vi "AMZ_S3_APIHLP_Parse Setup Bucket Notification Request Parameters.vi"(8 "error in (no error)":errorcluster, 11 "Setup Notification Request parameters":T1) -> (0 "error out":errorcluster, 5 "PUT Data":string)   [LabVIEW 2015, in "LV Interface for Amazon S3.lvlib"]
uses:
  LV Interface for Amazon S3.lvlib
  Typedefs/AMZ_S3_NotificationConfiguration.ctl
  Typedefs/AMZ_S3_CompleteTopicConfiguration.ctl
  Typedefs/AMZ_S3_Event.ctl
  Typedefs/AMZ_S3_FilterRule.ctl
  Typedefs/AMZ_S3_CloudFunctionConfiguration.ctl
  Typedefs/AMZ_S3_QueueConfiguration.ctl
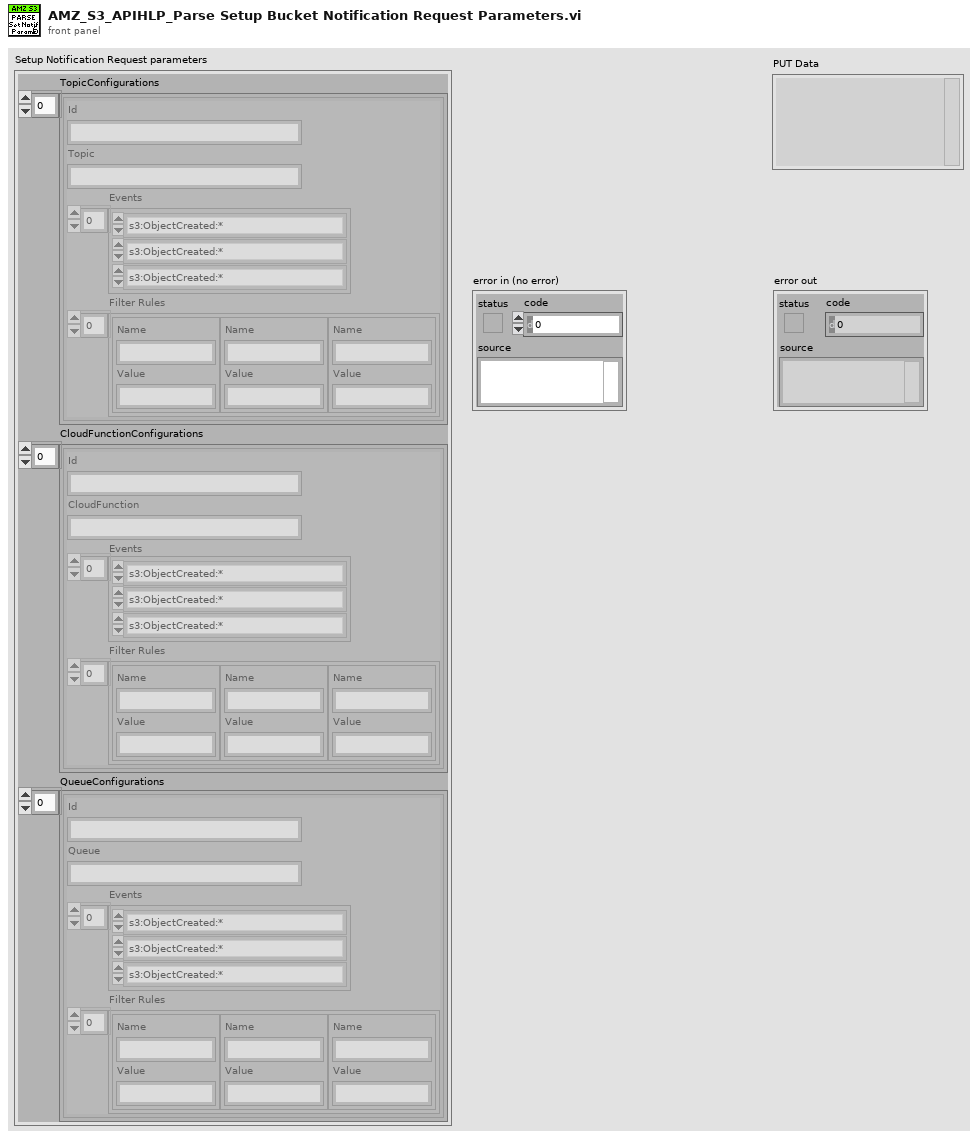
[diagram p1: front panel]
types:
  T1 = typedef "LV Interface for Amazon S3.lvlib/AMZ_S3_NotificationConfiguration.ctl" = cluster{"TopicConfigurations":T2[], "CloudFunctionConfigurations":T5[], "QueueConfigurations":T6[]}
  T2 = typedef "LV Interface for Amazon S3.lvlib/AMZ_S3_CompleteTopicConfiguration.ctl" = cluster{"Id":string, "Topic":string, "Events":T3[], "Filter Rules":T4[]}
  T3 = typedef "LV Interface for Amazon S3.lvlib/AMZ_S3_Event.ctl" = enum16{"s3:ObjectCreated:*", "s3:ObjectCreated:Put", "s3:ObjectCreated:Post", "s3:ObjectCreated:Copy", "s3:ObjectCreated:CompleteMultipartUpload", "s3:ObjectRemoved:*", "s3:ObjectRemoved:Delete", "s3:ObjectRemoved:DeleteMarkerCreated", "s3:ReducedRedundancyLostObject"}
  T4 = typedef "LV Interface for Amazon S3.lvlib/AMZ_S3_FilterRule.ctl" = cluster{"Name":string, "Value":string}
  T5 = typedef "LV Interface for Amazon S3.lvlib/AMZ_S3_CloudFunctionConfiguration.ctl" = cluster{"Id":string, "CloudFunction":string, "Events":T3[], "Filter Rules":T4[]}
  T6 = typedef "LV Interface for Amazon S3.lvlib/AMZ_S3_QueueConfiguration.ctl" = cluster{"Id":string, "Queue":string, "Events":T3[], "Filter Rules":T4[]}
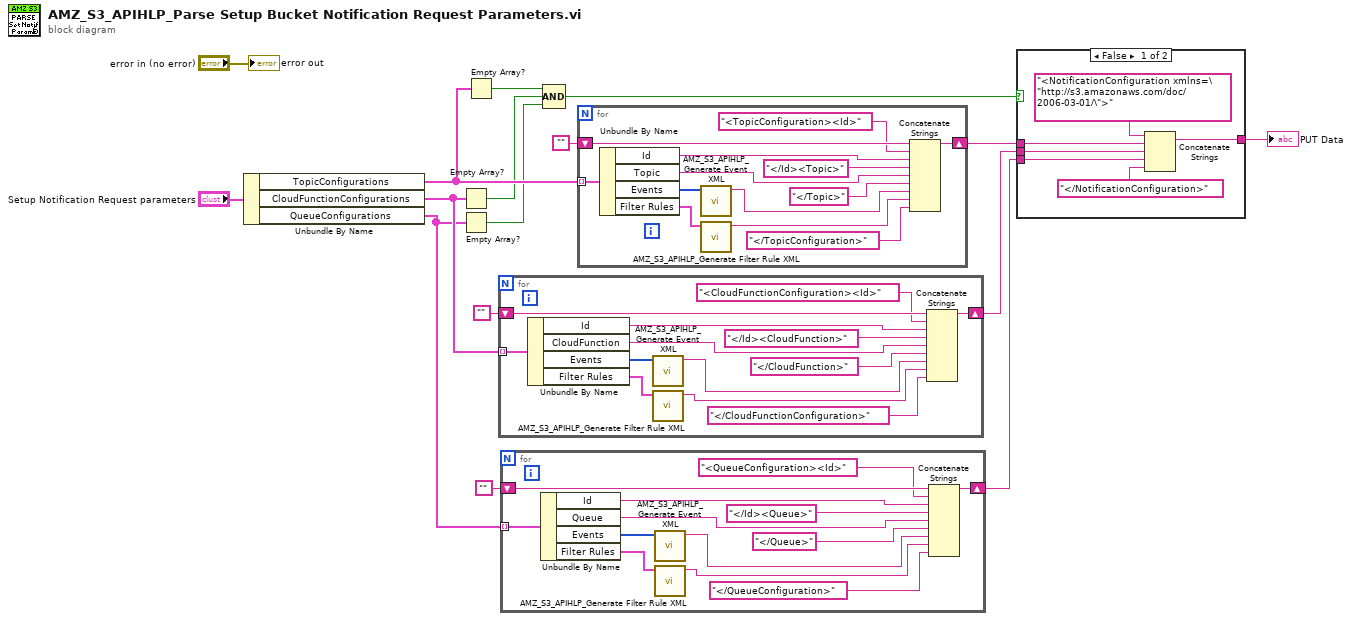
[diagram p0: block diagram]
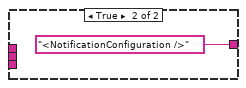
[diagram p2: hidden frame]
diagram:
  n1 = Unbundle By Name("Setup Notification Request parameters") -> ("TopicConfigurations"=w12:T2[], "CloudFunctionConfigurations"=w5:T5[], "QueueConfigurations"=w1:T6[])
  n2 = Empty Array?(array=w5) -> (empty?=w10:bool)
  n3 = Empty Array?(array=w1) -> (empty?=w9:bool)
  n4 = Empty Array?(array=w12) -> (empty?=w11:bool)
  n5 = for {
    tunnel: w5 -> [w26] mode=indexing
    shift-right: [w28] -> w4
    shift-left: "" -> [w29]
    n6 = Unbundle By Name(w26) -> ("Id"=w25:string, "CloudFunction"=w23:string, "Events"=w20:T3[], "Filter Rules"=w18:T4[])
    n7 = call "AMZ_S3_APIHLP_Generate Event XML.vi"("Events"=w20) -> ("Event XML"=w19:string)  [unwired: 10 in]
    n8 = call "AMZ_S3_APIHLP_Generate Filter Rule XML.vi"("Filter Rules"=w18) -> ("Filter Rule XML"=w17:string)  [unwired: 10 in]
    n9 = Concatenate Strings(w29, "<CloudFunctionConfiguration><Id>", w25, "</Id><CloudFunction>", w23, "</CloudFunction>", w19, w17, "</CloudFunctionConfiguration>") -> (w28:string)
  }
  n10 = for {
    tunnel: w1 -> [w39] mode=indexing
    shift-right: [w41] -> w2
    shift-left: "" -> [w42]
    n11 = Unbundle By Name(w39) -> ("Id"=w38:string, "Queue"=w36:string, "Events"=w33:T3[], "Filter Rules"=w31:T4[])
    n12 = call "AMZ_S3_APIHLP_Generate Event XML.vi"("Events"=w33) -> ("Event XML"=w32:string)  [unwired: 10 in]
    n13 = call "AMZ_S3_APIHLP_Generate Filter Rule XML.vi"("Filter Rules"=w31) -> ("Filter Rule XML"=w30:string)  [unwired: 10 in]
    n14 = Concatenate Strings(w42, "<QueueConfiguration><Id>", w38, "</Id><Queue>", w36, "</Queue>", w32, w30, "</QueueConfiguration>") -> (w41:string)
  }
  n15 = Compound Arithmetic op=AND(w11, w10, w9) -> (w8:bool)
  n16 = for {
    tunnel: w12 -> [w52] mode=indexing
    shift-right: [w54] -> w14
    shift-left: "" -> [w55]
    n17 = Unbundle By Name(w52) -> ("Id"=w51:string, "Topic"=w49:string, "Events"=w47:T3[], "Filter Rules"=w45:T4[])
    n18 = call "AMZ_S3_APIHLP_Generate Event XML.vi"("Events"=w47) -> ("Event XML"=w46:string)  [unwired: 10 in]
    n19 = call "AMZ_S3_APIHLP_Generate Filter Rule XML.vi"("Filter Rules"=w45) -> ("Filter Rule XML"=w44:string)  [unwired: 10 in]
    n20 = Concatenate Strings(w55, "<TopicConfiguration><Id>", w51, "</Id><Topic>", w49, "</Topic>", w46, w44, "</TopicConfiguration>") -> (w54:string)
  }
  n21 = case shown="False" w8 {
    tunnel: w14 -> [w61 _]
    tunnel: [w60 "<NotificationConfiguration />"] -> w13
    tunnel: w4 -> [w58 _]
    tunnel: w2 -> [w56 _]
    frame False {
      n22 = Concatenate Strings("<NotificationConfiguration xmlns=\"http://s3.amazonaws.com/doc/2006-03-01/\">", w61, w58, w56, "</NotificationConfiguration>") -> (w60:string)
    }
    frame True {
    }
  }
  "PUT Data" <- w13
  "error out" <- "error in (no error)"
